vi "From Serial Form.vi"(6 "Serial Version":T1, 10 "Deserializer in":refnum<class "Deserializer.lvclass">, 11 "BrowerComposite in":refnum<class "BrowerComposite.lvclass">) -> (0 "error out":errorcluster, 2 "Deserializer out":refnum<class "Deserializer.lvclass">, 3 "BrowerComposite out":refnum<class "BrowerComposite.lvclass">)   [LabVIEW 2015, in "BrowerComposite.lvclass"]
uses:
  BrowerComposite.lvclass
  <vilib>/NI/AQ Character Lineator/Deserializer/Deserializer.lvclass
  <vilib>/NI/AQ Character Lineator/Serialization Common/Serial Version.ctl
  <vilib>/NI/AQ Character Lineator/Serializable/Remove Serializable Array.vi
  <vilib>/NI/AQ Character Lineator/Serializable/Remove String Array.vi
  <vilib>/NI/AQ Character Lineator/Serializable/Remove Serializable.vi
  BrowerComponent/BrowerComponent.lvclass
  <vilib>/NI/AQ Character Lineator/Serializable/Serializable.lvclass
  <vilib>/NI/AQ Character Lineator/Serialization Common/Serialization Common.lvlib
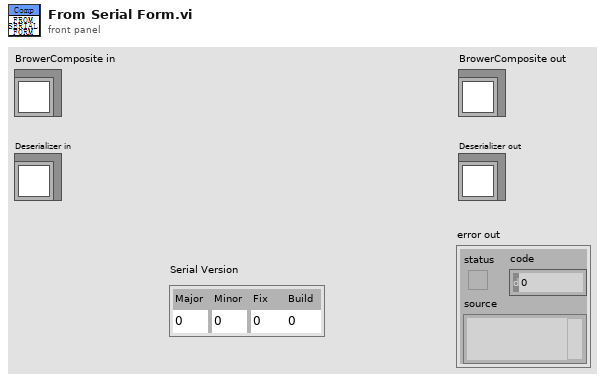
[diagram p1: front panel]
types:
  T1 = typedef "Serialization Common.lvlib/Serial Version.ctl" = cluster{"Major":u16, "Minor":u16, "Fix":u16, "Build":u16}
  T2 = typedef "BrowerComposite.lvclass/ObjectAttributes.ctl" = cluster{"BrowerComponents":refnum<class "BrowerComponent.lvclass">[], "BrowerComponentIDs":string[], "Iterator":refnum<class "Iterator.lvclass">}
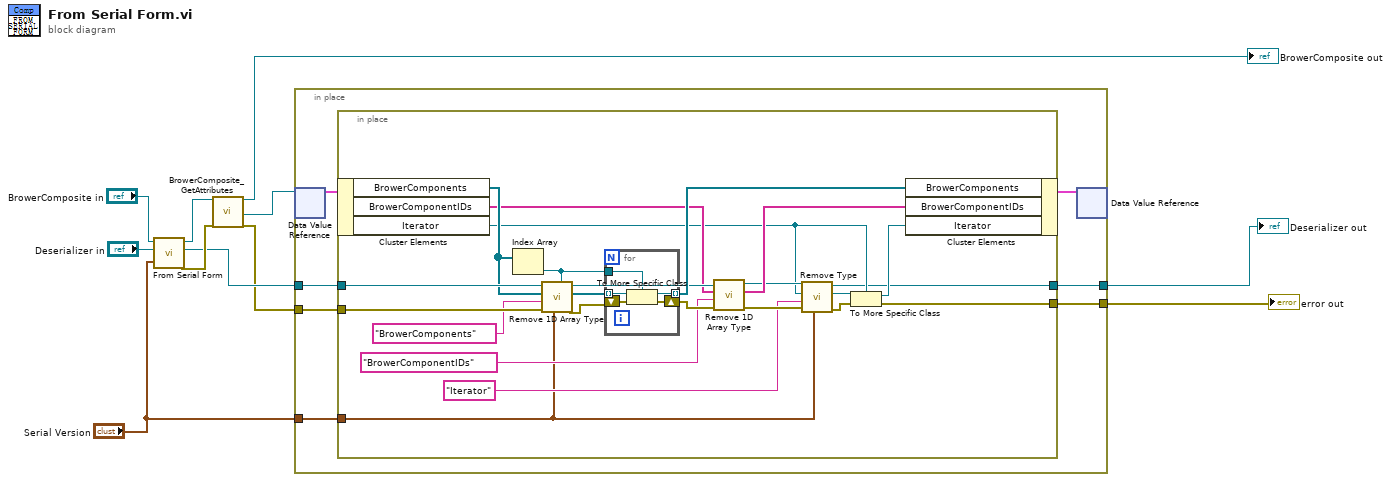
[diagram p0: block diagram]
diagram:
  n1 = call-parent "From Serial Form.vi"("Serial Version"="Serial Version", "Deserializer in"="Deserializer in", "BrowerComponent in"="BrowerComposite in") -> ("error out"=w9:errorcluster, "Deserializer out"=w6:refnum<class "Deserializer.lvclass">, "BrowerComponent out"=w8:refnum<class "BrowerComposite.lvclass">)  [unwired: 6 in]
  n2 = call "BrowerComposite_GetAttributes.vi"("reference in"=w8, "error in (no error)"=w9) -> ("reference out"=→"BrowerComposite out":refnum<class "BrowerComposite.lvclass">, "DataRef"=w7:refnum<data-value>, "error out"=w5:errorcluster)  [unwired: 14 in, 1 out]
  n3 = in-place {
    in-place-border: w6 -> [w18]
    in-place-border: w5 -> [w16]
    in-place-border: [w14] -> w4
    in-place-border: [w13] -> w3
    in-place-border: "Serial Version" -> [w12]
    n4 = in-place-dvr #1(w7) -> (w17:T2)  [unwired: 1 out]
    n5 = in-place {
      in-place-border: w18 -> [w41]
      in-place-border: w16 -> [w38]
      in-place-border: [w21] -> w14
      in-place-border: [w20] -> w13
      in-place-border: w12 -> [w19]
      n6 = in-place-cluster #2(w17) -> ("BrowerComponents"=w40:refnum<class "BrowerComponent.lvclass">[], "BrowerComponentIDs"=w32:string[], "Iterator"=w24:refnum<class "Iterator.lvclass">)
      n7 = Index Array(array=w40) -> (element=w36:refnum<class "BrowerComponent.lvclass">)  [unwired: 1 in]
      n8 = call-poly <vilib>:"Remove 1D Array Type.vi"("Default Serializable Type"=w36, "Serial Version"=w19, "error in (no error)"=w38, "Name"="BrowerComponents", "Default Value"=w40, "Deserializer in"=w41) -> ("error out"=w37:errorcluster, "Serializables"=w39:refnum<class "Serializable.lvclass">[], "Deserializer out"=w34:refnum<class "Deserializer.lvclass">)  [unwired: 2 in, 1 out]
      n9 = for {
        tunnel: w39 -> [w46] mode=indexing
        shift-right: [w44] -> w33
        shift-left: w37 -> [w45]
        tunnel: [w43] -> w35 mode=indexing
        tunnel: w36 -> [w42]
        n10 = To More Specific Class(target class=w42, reference=w46, error in=w45) -> (specific class reference=w43:refnum<class "BrowerComponent.lvclass">, error out=w44:errorcluster)
      }
      n11 = call-poly <vilib>:"Remove 1D Array Type.vi"("error in (no error)"=w33, "Name"="BrowerComponentIDs", "Default Value"=w32, "Deserializer in"=w34) -> ("error out"=w29:errorcluster, "Strings"=w31:string[], "Deserializer out"=w30:refnum<class "Deserializer.lvclass">)  [unwired: 4 in, 1 out]
      n12 = call-poly <vilib>:"Remove Type.vi"("Serial Version"=w19, "error in (no error)"=w29, "Name"="Iterator", "Default Value"=w24, "Deserializer in"=w30) -> ("error out"=w23:errorcluster, "Serializable"=w25:refnum<class "Serializable.lvclass">, "Deserializer out"=w20:refnum<class "Deserializer.lvclass">)  [unwired: 3 in, 1 out]
      n13 = To More Specific Class(target class=w24, reference=w25, error in=w23) -> (specific class reference=w22:refnum<class "Iterator.lvclass">, error out=w21:errorcluster)
      n14 = in-place-cluster #2("BrowerComponents"=w35, "BrowerComponentIDs"=w31, "Iterator"=w22) -> (w15:T2)
    }
    n15 = in-place-dvr #1(w15) -> ()  [unwired: 2 out]
  }
  "error out" <- w4
  "Deserializer out" <- w3
